vi "例程08-计算平方和.vi"() -> ()   [LabVIEW 2016]
panel:
  in  "停止":bool
  out "平方和":string
  in  "输入n":i32
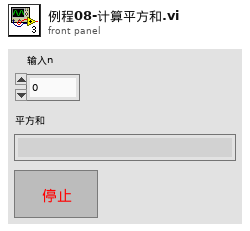
[diagram p1: front panel]
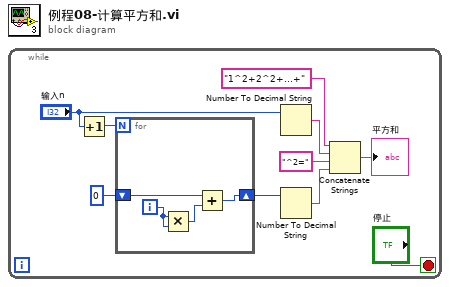
[diagram p0: block diagram]
diagram:
  n1 = while {
    stop <- "停止" stop-if-true
    n2 = Increment(x="输入n") -> (x+1=w10:i32)
    n3 = for {
      N: w10 -> [_]
      shift-right: [w11] -> w8
      shift-left: 0 -> [w13]
      i -> [w14]
      n4 = Multiply(x=w14, y=w14) -> (x*y=w12:i32)
      n5 = Add(x=w13, y=w12) -> (x+y=w11:i32)
    }
    n6 = Number To Decimal String(number="输入n") -> (decimal integer string=w4:string)  [unwired: 1 in]
    n7 = Number To Decimal String(number=w8) -> (decimal integer string=w2:string)  [unwired: 1 in]
    n8 = Concatenate Strings("1^2+2^2+...+" ("字符串"), w4, "^2=" ("字符串"), w2) -> (→"平方和":string)
  }
